vi "SQL_Alarm_condition.vi"   [LabVIEW 2014]
uses:
  Terminal_Global_Alarm_condition.vi
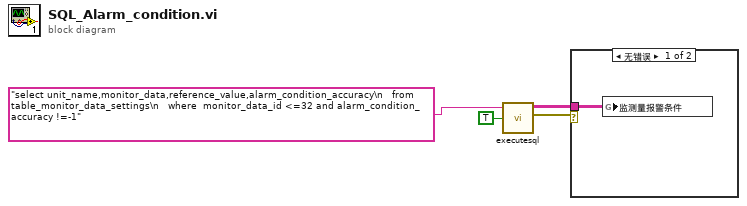
[diagram p0: block diagram]
diagram:
  n1 = call "executesql.vi"("Return Data (T)"=TRUE, "Command Text"="select unit_name,monitor_data,reference_value,alarm_condition_accuracy\n   from table_monitor_data_settings\n   where  monitor_data_id <=32 and alarm_condition_accuracy !=-1") -> ("error out"=w2:errorcluster, "Data"=w1:string[][])  [unwired: 5 in]
  n2 = case shown="无错误" w2 {
    tunnel: w1 -> [w5 _]
    frame No Error {
      n3 = global write "Terminal_Global_Alarm_condition.vi" "监测量报警条件"(w5) -> ()
    }
    frame Error {
    }
  }
